vi "Type Conversion.From Double (I32).vi"(3 "value in":dbl) -> (1 "value out":i32)   [LabVIEW 2016, in "VeriStand Data.lvlib"]
doc: "Converts the provided double float values to the specified data type, preserving the numerical value of the data."
uses:
  VeriStand Data.lvlib
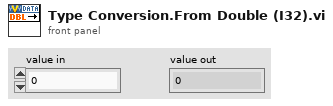
[diagram p1: front panel]
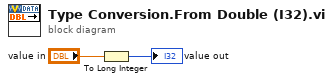
[diagram p0: block diagram]
diagram:
  n1 = To Long Integer(number="value in") -> (32bit integer=→"value out":i32)
